vi "MoveSnakes.vi"(8 "error in (no error)":errorcluster, 10 "Engine in":refnum<class "Engine.lvclass">, 11 "Pong in":refnum<class "Pong.lvclass">) -> (0 "error out":errorcluster, 2 "Engine out":refnum<class "Engine.lvclass">, 3 "Pong out":refnum<class "Pong.lvclass">)   [LabVIEW 2019, in "RT_Game.lvlib" / "Pong.lvclass"]
uses:
  Pong.lvclass
  C:/Users/FreshBob/Dropbox/VIs/myRIO_GameConsole/RT/RT_Game/Game/Game.lvclass
  Engine/Engine.lvclass
  Game/Game.lvclass/Game.ctl
  Pong.lvclass/Pong.ctl
  Engine/Engine.lvclass/Engine.ctl
  Game/Read Singleplayer.vi
  Read pause_time.vi
  PongPanel/PongPanel.lvclass
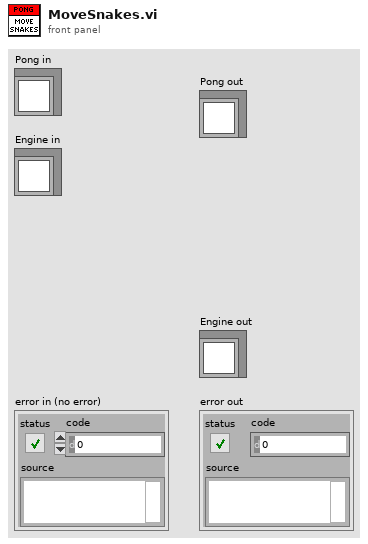
[diagram p1: front panel]
types:
  T1 = typedef "RT_Game.lvlib/Engine.lvclass/Controls.ctl" = cluster{"Controls_1":T2, "Controls_2":cluster{"DirectionX":i8, "DirectionY":i8, "Button1":bool, "Button2":bool}, "SystemButton":bool}
  T2 = typedef "RT_Game.lvlib/Engine.lvclass/ControlPlayer.ctl" = cluster{"DirectionX":i8, "DirectionY":i8, "Button1":bool, "Button2":bool}
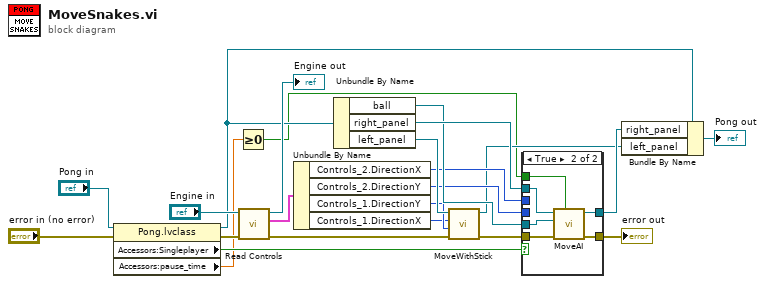
[diagram p0: block diagram]
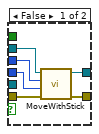
[diagram p2: hidden frame]
diagram:
  n1 = property class="Pong.lvclass"(reference="Pong in", error in="error in (no error)") -> (reference out=w4:refnum<class "Pong.lvclass">, error out=w6:errorcluster, "Accessors:Singleplayer"=w3:bool, "Accessors:pause_time"=w2:dbl)
  n2 = Greater Or Equal To 0?(x=w2) -> (x >= 0?=w1:bool)
  n3 = call "Read Controls.vi"("error in (no error)"=w6, "Engine in"="Engine in") -> ("error out"=w19:errorcluster, "Controls"=w21:T1, "Engine out"=→"Engine out":refnum<class "Engine.lvclass">)  [unwired: 7 in]
  n4 = Unbundle By Name(w21) -> ("Controls_2.DirectionX"=w11:i8, "Controls_2.DirectionY"=w12:i8, "Controls_1.DirectionY"=w10:i8, "Controls_1.DirectionX"=w9:i8)
  n5 = Unbundle By Name(w4) -> ("ball"=w16:refnum<class "PongBall.lvclass">, "right_panel"=w17:refnum<class "PongPanel.lvclass">, "left_panel"=w18:refnum<class "PongPanel.lvclass">)
  n6 = call "MoveWithStick.vi"("error in (no error)"=w19, "DirectionY"=w10, "DirectionX"=w9, "PongPanel in"=w18) -> ("error out"=w14:errorcluster, "PongPanel out"=w7:refnum<class "PongPanel.lvclass">)  [unwired: 6 in]
  n7 = case shown="True" w3 {
    tunnel: [w29 w34] -> w13
    tunnel: [w28 w32] -> w8
    tunnel: w12 -> [w27 _]
    tunnel: w11 -> [w26 _]
    tunnel: w14 -> [w25 w35]
    tunnel: w17 -> [w24 w33]
    tunnel: w16 -> [_ w31]
    tunnel: w1 -> [_ w30]
    frame False {
      n8 = call "MoveWithStick.vi"("error in (no error)"=w25, "DirectionY"=w27, "DirectionX"=w26, "PongPanel in"=w24) -> ("error out"=w29:errorcluster, "PongPanel out"=w28:refnum<class "PongPanel.lvclass">)  [unwired: 6 in]
    }
    frame True {
      n9 = call-dynamic "MoveAI.vi"("ReturnHome(F)"=w30, "error in (no error)"=w35, "Ball"=w31, "PongPanel in"=w33) -> ("error out"=w34:errorcluster, "PongPanel out"=w32:refnum<class "PongPanel.lvclass">)  [unwired: 6 in]
    }
  }
  "error out" <- w13
  n10 = Bundle By Name(cluster=w4, "right_panel"=w8, "left_panel"=w7) -> (→"Pong out":refnum<class "Pong.lvclass">)
